vi "Agilent DMM Configure Serial Port.vi"(8 "error in (no error)":errorcluster, 11 "VISA Resource Name":refnum<visa-resource-name>) -> (0 "error out":errorcluster, 3 "dup VISA Resource Name":refnum<visa-resource-name>)   [LabVIEW 2011]
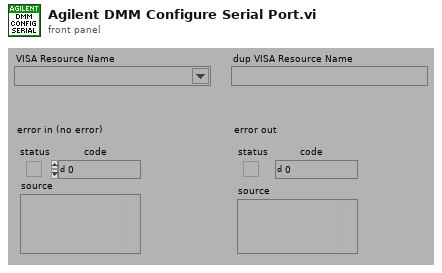
[diagram p1: front panel]
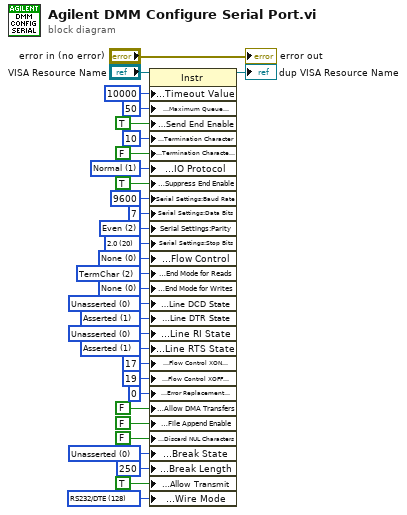
[diagram p0: block diagram]
diagram:
  w29 = i16 128 items=["Unknown"=-1, "RS485/Wire4"=0, "RS485/Wire2-EchoDTR"=1, "RS485/Wire2-CtrlDTR"=2, "RS485/Wire2-Auto"=3, "RS232/DTE"=128, "RS232/DCE"=129, "RS232/AUTO"=130] ("Serial Settings:Wire Mode")
  w26 = i16 0 items=["Unknown"=-1, "Unasserted"=0, "Asserted"=1] ("Modem Line Settings:Break State")
  w19 = i16 1 items=["Unknown"=-1, "Unasserted"=0, "Asserted"=1] ("Modem Line Settings:Line RTS State")
  w18 = i16 0 items=["Unknown"=-1, "Unasserted"=0, "Asserted"=1] ("Modem Line Settings:Line RI State")
  w17 = i16 1 items=["Unknown"=-1, "Unasserted"=0, "Asserted"=1] ("Modem Line Settings:Line DTR State")
  w16 = i16 0 items=["Unknown"=-1, "Unasserted"=0, "Asserted"=1] ("Modem Line Settings:Line DCD State")
  w15 = u16 0 items=["None", "LastBit", "TermChar", "Break"] ("Serial Settings:Serial End Mode for Writes")
  w14 = u16 2 items=["None", "LastBit", "TermChar"] ("Serial Settings:Serial End Mode for Reads")
  w13 = u16 0 items=["None", "XON/XOFF", "RTS/CTS", "XON/XOFF & RTS/CTS", "DTR/DSR", "XON/XOFF & DTR/DSR"] ("Serial Settings:Serial Flow Control")
  w12 = u16 20 items=["1.0"=10, "1.5"=15, "2.0"=20] ("Serial Settings:Serial Stop Bits")
  w11 = u16 2 items=["None", "Odd", "Even", "Mark", "Space"] ("Serial Settings:Serial Parity")
  w8 = u16 1 items=["Normal"=1, "VXI/FDC"=2, "GPIB/HS488"=3, "Serial-TCPIP-USB/488-Strings"=4, "USBTMC/Vendor-Specific"=5] ("Message Based Settings:IO Protocol")
  n1 = property class="Instr"(reference="VISA Resource Name", "General Settings:Timeout Value"=u32 10000, "General Settings:Maximum Queue Length"=u32 50, "Message Based Settings:Send End Enable"=TRUE, "Message Based Settings:Termination Character"=u8 10, "Message Based Settings:Termination Character Enable"=FALSE, "Message Based Settings:IO Protocol"=w8, "Message Based Settings:Suppress End Enable"=TRUE, "Serial Settings:Baud Rate"=u32 9600 ("Serial Settings:Serial Baud Rate"), "Serial Settings:Data Bits"=u16 7 ("Serial Settings:Serial Data Bits"), "Serial Settings:Parity"=w11, "Serial Settings:Stop Bits"=w12, "Serial Settings:Flow Control"=w13, "Serial Settings:End Mode for Reads"=w14, "Serial Settings:End Mode for Writes"=w15, "Serial Settings:Modem Line Settings:Line DCD State"=w16, "Serial Settings:Modem Line Settings:Line DTR State"=w17, "Serial Settings:Modem Line Settings:Line RI State"=w18, "Serial Settings:Modem Line Settings:Line RTS State"=w19, "Serial Settings:Flow Control XON Character"=u8 17, "Serial Settings:Flow Control XOFF Character"=u8 19, "Serial Settings:Error Replacement Character"=u8 0, "General Settings:Allow DMA Transfers"=FALSE, "Message Based Settings:File Append Enable"=FALSE, "Serial Settings:Discard NUL Characters"=FALSE, "Serial Settings:Modem Line Settings:Break State"=w26, "Serial Settings:Break Length"=i16 250, "Serial Settings:Allow Transmit"=TRUE, "Serial Settings:Wire Mode"=w29) -> (reference out=→"dup VISA Resource Name":refnum<visa-resource-name>)  [unwired: 1 in, 1 out]
  "error out" <- "error in (no error)"
